vi "nidaq_Analog_Output_Vi.vi"(1 "start Solenoide Valve":bool caption="start chromat", 2 "start chromat":bool) -> ()   [LabVIEW 2011]
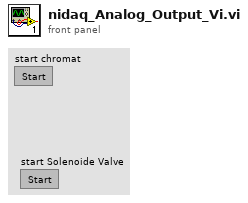
[diagram p1: front panel]
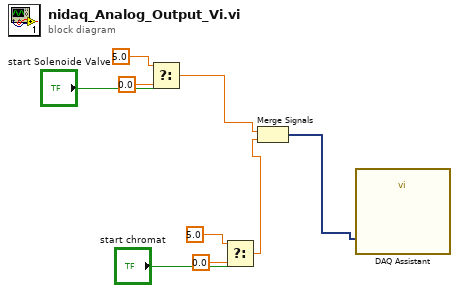
[diagram p0: block diagram]
diagram:
  n1 = Select(t=5.0, s="start Solenoide Valve", f=0.0) -> (s? t:f=w1:dbl)
  n2 = Select(t=5.0, s="start chromat", f=0.0) -> (s? t:f=w5:dbl)
  n3 = Merge Signals(w1, w5) -> (w6:dynamicdata)
  n4 = call "DAQ Assistant"("data"=w6) -> ()  [unwired: 17 in, 2 out]
